vi "Oscilloscope_old.vi"(6 "Slow Control User":string, 9 "notifier in":T4, 10 "queue in":T3) -> ()   [LabVIEW 2012]
uses:
  Oscilloscope/TypeDefs/DataTypes/OscilloscopeState.ctl
  Oscilloscope/TypeDefs/Paths/DataPath.ctl
  <vilib>/Analysis/NI_AALPro.lvlib
  Oscilloscope/TypeDefs/DataTypes/Data.ctl
  TypeDefs/DataTypes/SystemStatus.ctl
  Oscilloscope/TypeDefs/DataTypes/RunInfo.ctl
  Oscilloscope/TypeDefs/DataTypes/UIReferences.ctl
  Oscilloscope/TypeDefs/DataTypes/Measurement.ctl
  Oscilloscope/TypeDefs/DataTypes/Acquisition.ctl
  Oscilloscope/TypeDefs/DataTypes/StopCondition.ctl
  Oscilloscope/TypeDefs/DataTypes/Current.ctl
  Oscilloscope/TypeDefs/DataTypes/DAQConfig.ctl
  <vilib>/Utility/xml.llb/Read From XML File(string).vi
  <vilib>/Analysis/6fits.llb/Remove Outliers (Range).vi
  TypeDefs/QueueNotifier/DataQueue.ctl
  TypeDefs/QueueNotifier/Notifier.ctl
  Oscilloscope/TypeDefs/DataTypes/AcquisitionInfo.ctl
panel:
  in  "SaveToggle":bool caption="Stop Condition"
  in  "Acquisition Info":T1 {"Shaping Amplifier" items=["CR-200-1us", "CR-200-100ns", "", ""]; "Preamplifier" items=["CR-Z-113-1k", "CR-Z-113-5k", "CR-Z-SiPM", ""]}
  out "Acquisition Rate":dbl format="%#.1f"
  in  "Stop":bool
  in  "View TDMS":bool caption="Configure DAQ"
  in  "Trigger Level (V)":dbl=-0.02
  in  "Range (V)":dbl(ring)=2.0 items=["10"=10.0, "5"=5.0, "2"=2.0, "1"=1.0, "0.4"=0.4, "0.2"=0.2, "0.08"=0.08, "0.04"=0.04, "0.02"=0.02, "0.01"=0.01]
  in  "Offset (V)":dbl=-0.5
  out "Acquiring Now?":bool
  out "Active Run?":bool
  out "Time Elapsed (s)":dbl format="%#.1f"
  out "Waveforms Acquired":dbl
  in  "Stop Condition":T2={"Quota"=2000.0, "Duration (S)"=120, "Stop Condition"=FALSE}
  in  "Run Info":bool caption="Configure DAQ"
  out "Signal":waveform(dbl)(graph)
  in  "Measurement (Ch1)":i32(ring)=26 items=["AC RMS"=1, "Amplitude"=2, "Average"=3, "Cycle Average"=4, "Cycle Frequency"=5, "Cycle Period"=6, "Cycle RMS"=7, "DC RMS"=8, "Estimated Number of Bits"=9, "Falling Edges"=10, "Fall Overshoot"=11, "Fall Preshoot"=12, "Frequency"=13, "Fall Crossing Time"=14, "Fall Time"=15, "High"=16, "Low"=17, "Maximum"=18, "Minimum"=19, "Mid"=20, "Negative Duty"=21, "Negative Width"=22, "Positive Duty"=23, "Period"=24, "Phase"=25, "Peak to Peak"=26, "Positive Width"=27, "Rising Edges"=28, "Rise Overshoot"=29, "Rise Preshoot"=30, "Rise Crossing Time"=31, "Rise Time"=32, "Standard Deviation"=33, "Spurious Free Dynamic Range"=34, "Signal to Noise+Distortion"=35, "Signal to Noise"=36, "Total Harmonic Distortion"=37, "Time of Maximum"=38, "Time of Minimum"=39]
  in  "New Run":bool caption="Configure DAQ"
  in  "Export":bool caption="Configure DAQ"
  in  "Exit":bool caption="Configure DAQ"
  in  "Save Run":bool caption="Configure DAQ"
  in  "Settings":bool caption="Configure DAQ"
  in  "Acquire":bool
  out "Preliminary Histogram":cluster{"Y":dbl[], "Y":dbl[]}[](graph)
  # "Shaper Gain"
  # "Self"
  # "Fast"
  # "Solicited"
  # "Standard"
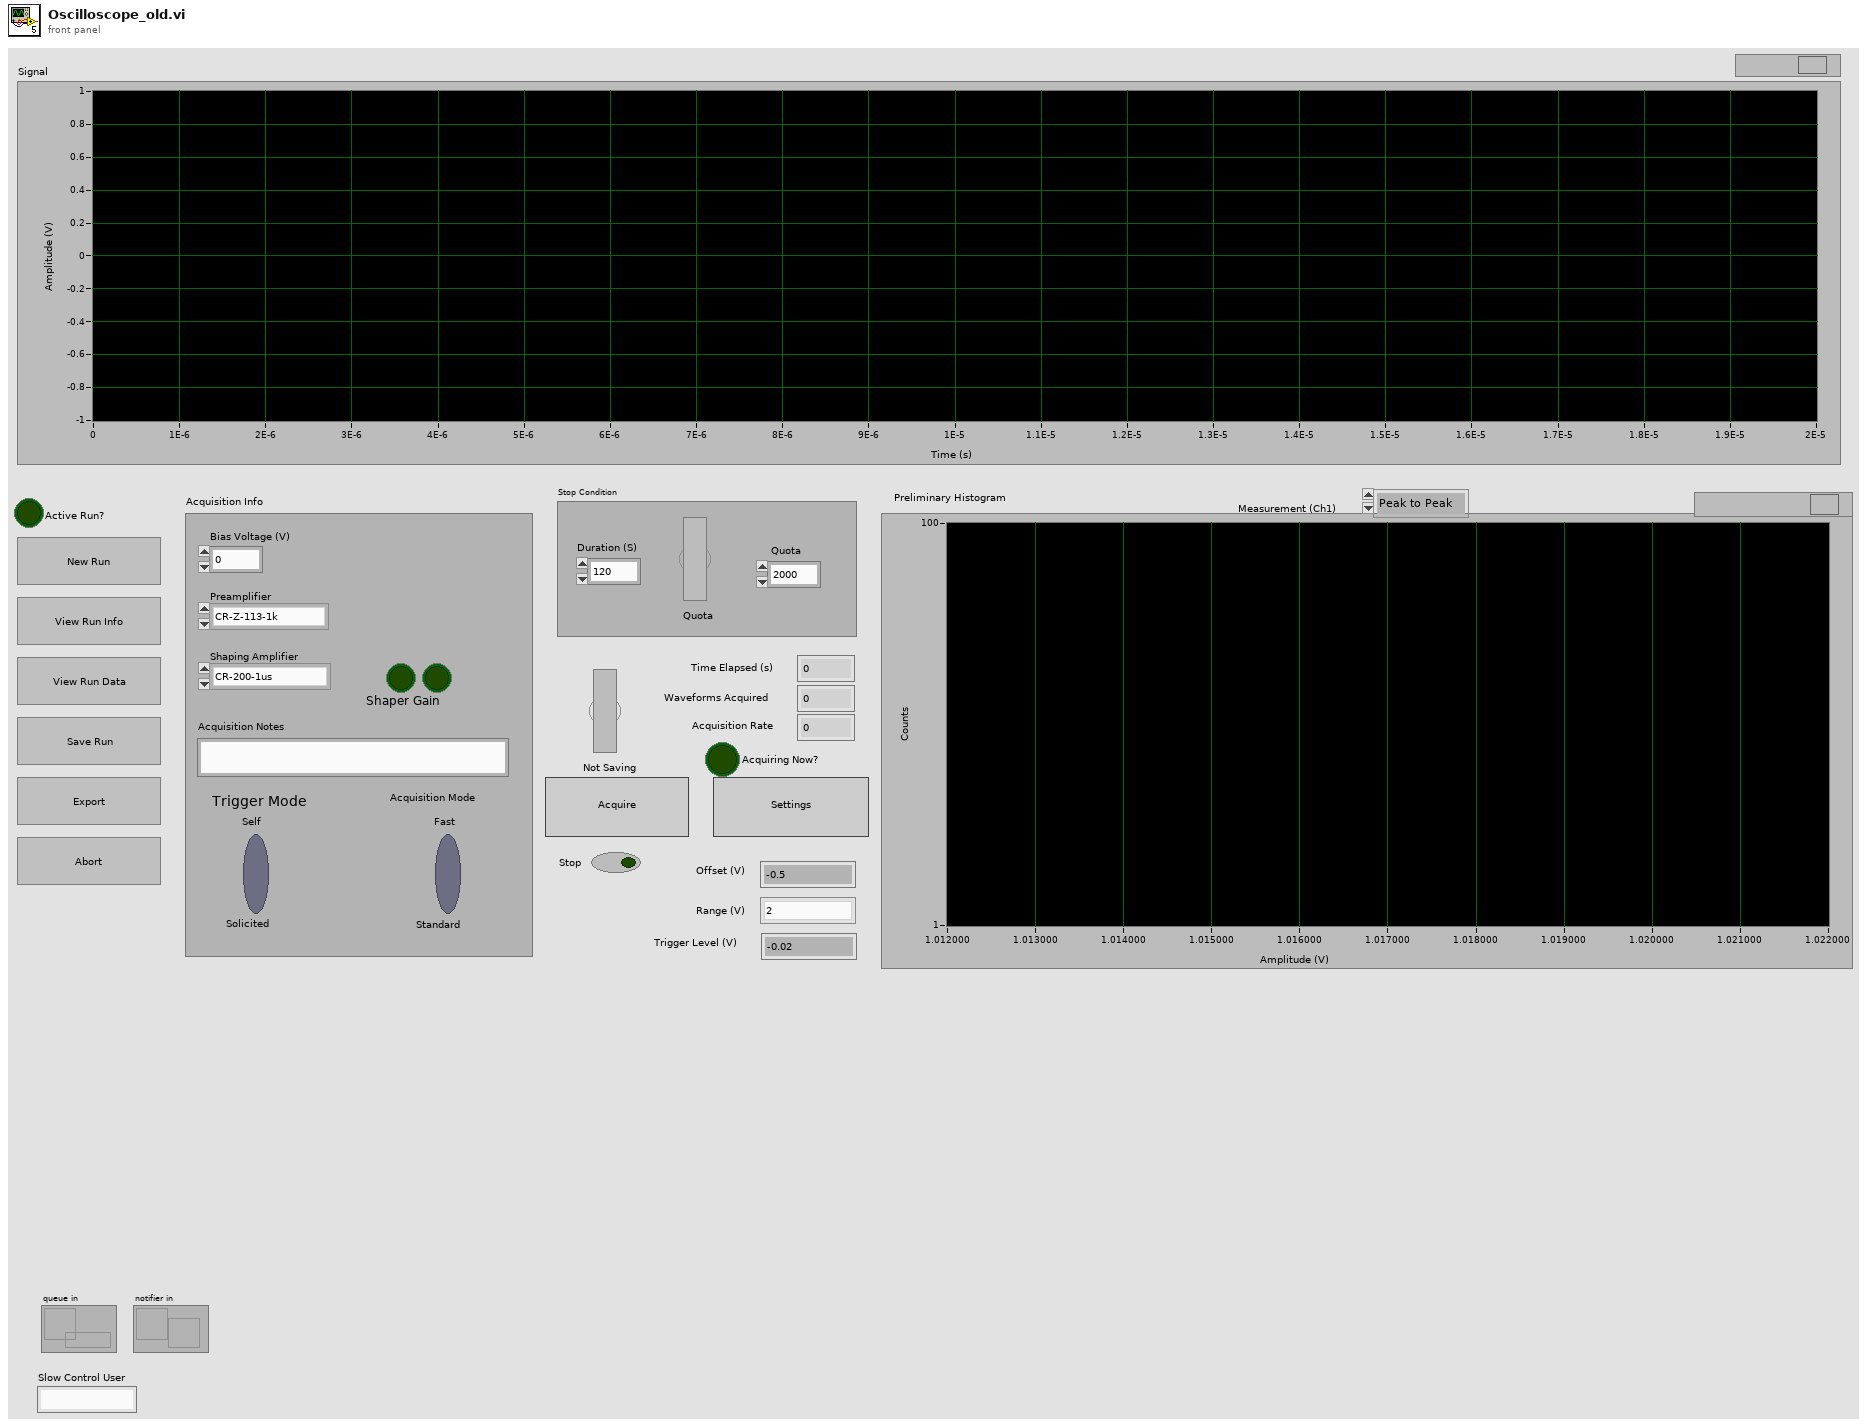
[diagram p1: front panel]
types:
  T1 = typedef "AcquisitionInfo.ctl" = cluster{"Trigger Mode":bool, "Acquisition Mode":bool, "Bias Voltage (V)":dbl, "Preamplifier":u16, "Shaping Amplifier":u16, "Acquisition Notes":string, "1":bool, "2":bool}
  T2 = typedef "StopCondition.ctl" = cluster{"Quota":dbl, "Duration (S)":u16, "Stop Condition":bool}
  T3 = typedef "DataQueue.ctl" = refnum<queue>
  T4 = typedef "Notifier.ctl" = refnum<notifier>
  T5 = typedef "DataPath.ctl" = path
  T6 = typedef "Data.ctl" = cluster{"DAQ Config Data":T7, "Acquisition":T8, "Measurement":T10, "UI References":T11, "Run Info":T12, "System Status":T13, "Acquisition Info":cluster{"Trigger Mode":bool, "Acquisition Mode":bool, "Bias Voltage (V)":dbl, "Preamplifier":u16, "Shaping Amplifier":u16, "Acquisition Notes":string, "1":bool, "2":bool}}
  T7 = typedef "DAQConfig.ctl" = cluster{"Vertical":cluster{"Coupling":i32, "Offset (V)":dbl, "Range (V)":dbl, "Impedance":dbl}, "Horizontal":cluster{"Offset Time":dbl, "Sample Time (S)":dbl, "Sample Points":u32}, "Trigger\n":cluster{"Lower Level (V)":dbl, "Trigger Slope":i32, "Trigger Source":i32}, "Acquisition":cluster{"Trigger Mode":i32, "Initiate Continuously":i32, "Acquire Type":i32, "Acquire Count":i32}, "Channel":i32, "Instrument Handle":i32, "Error":errorcluster, "State":i32}
  T8 = typedef "Acquisition.ctl" = cluster{"Current":T9, "Stop Condition":T2, "Config Needed":bool}
  T9 = typedef "Current.ctl" = cluster{"Acquiring Now?":bool, "Waveforms Acquired":dbl, "Start of Acquisition":timestamp, "Acquisition Name":string}
  T10 = typedef "Measurement.ctl" = cluster{"Waveform":waveform(dbl), "Peak Heights":dbl[], "Acquisition Time":timestamp, "File Path":path, "TDMS File Handle":refnum<k34>}
  T11 = typedef "UIReferences.ctl" = cluster{"Acquire":refnum<vi>, "Configure DAQ":refnum<vi>, "Measurement (Ch1)":refnum<vi>, "Update Needed?":bool, "New Run":refnum<vi>, "Signal":refnum<vi>}
  T12 = typedef "RunInfo.ctl" = cluster{"Active Run?":bool, "Run Notes":string, "User Name":string, "Campaign ID#":string, "Run Name":string, "Start Time":timestamp, "End Time":timestamp}
  T13 = typedef "SystemStatus.ctl" = cluster{"Bias Voltage":dbl, "SiPM Temperature":dbl[], "Slow Control User":string, "LXe":dbl}
  T14 = typedef "OscilloscopeState.ctl" = enum16{"Acquire", "Initialize", "Waiting For Event", "New Run", "Settings", "Update UI", "ViewRunInfo", "Synchronize", "Fast Acquire"}
  T15 = enum8{"Enabled", "Disabled", "Disabled and Grayed Out"}
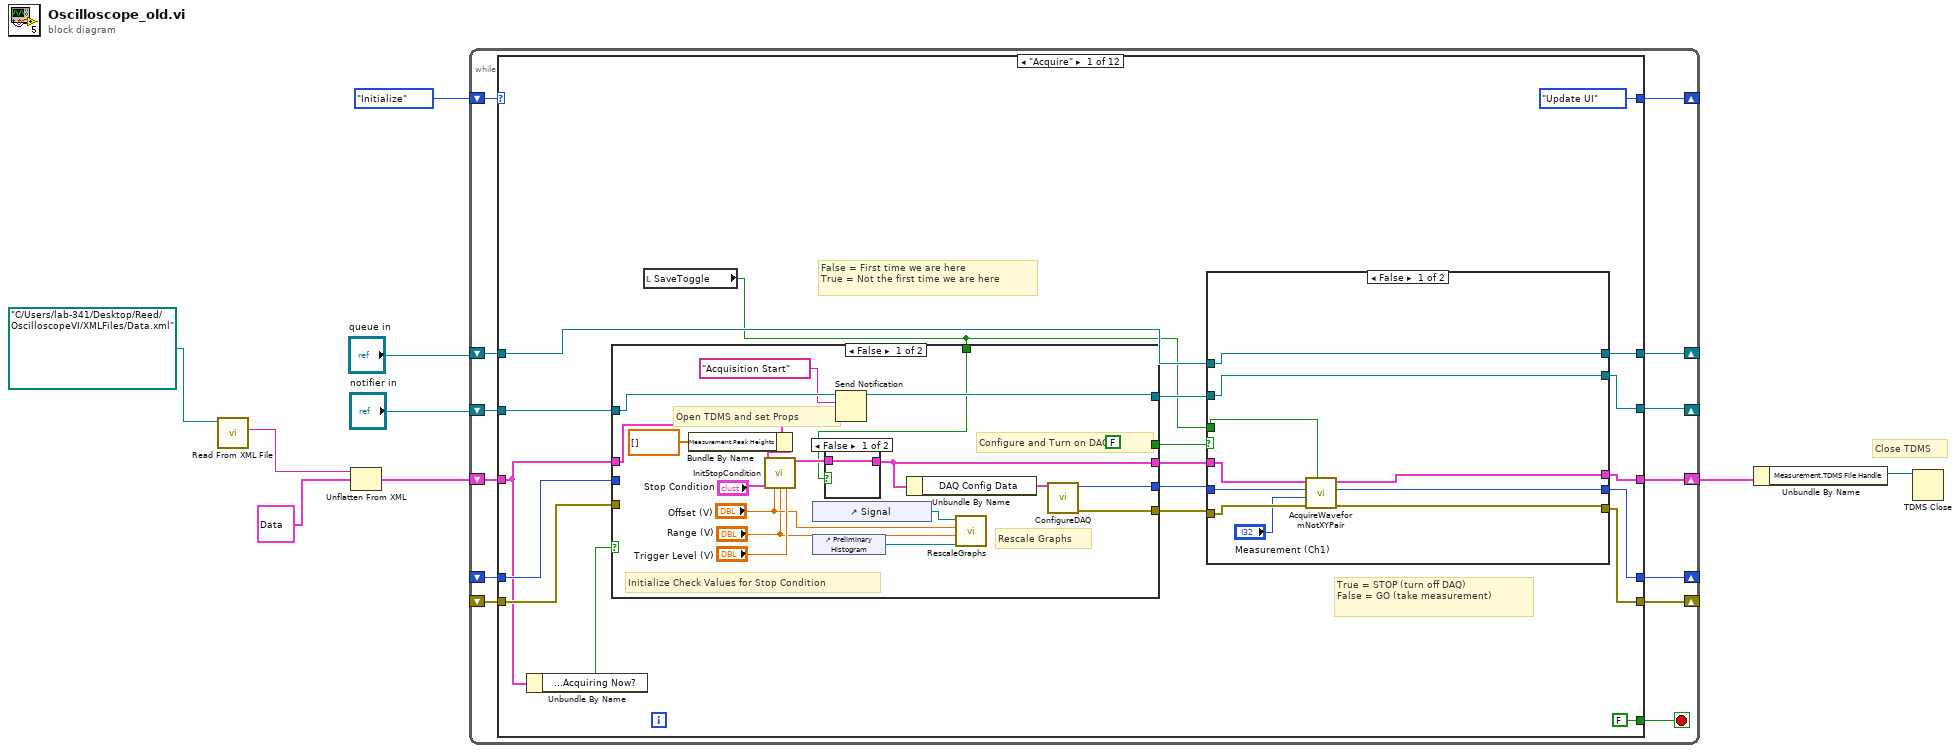
[diagram p0: block diagram]
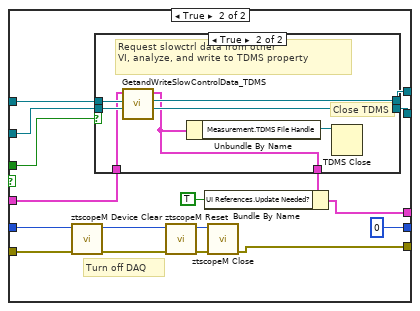
[diagram p2: hidden frame]
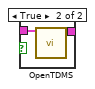
[diagram p4: hidden frame]
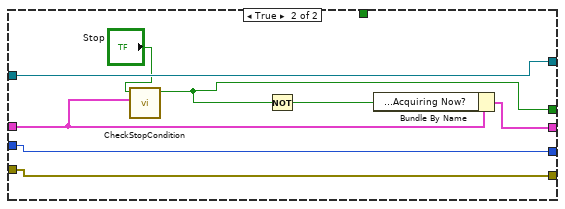
[diagram p5: hidden frame]
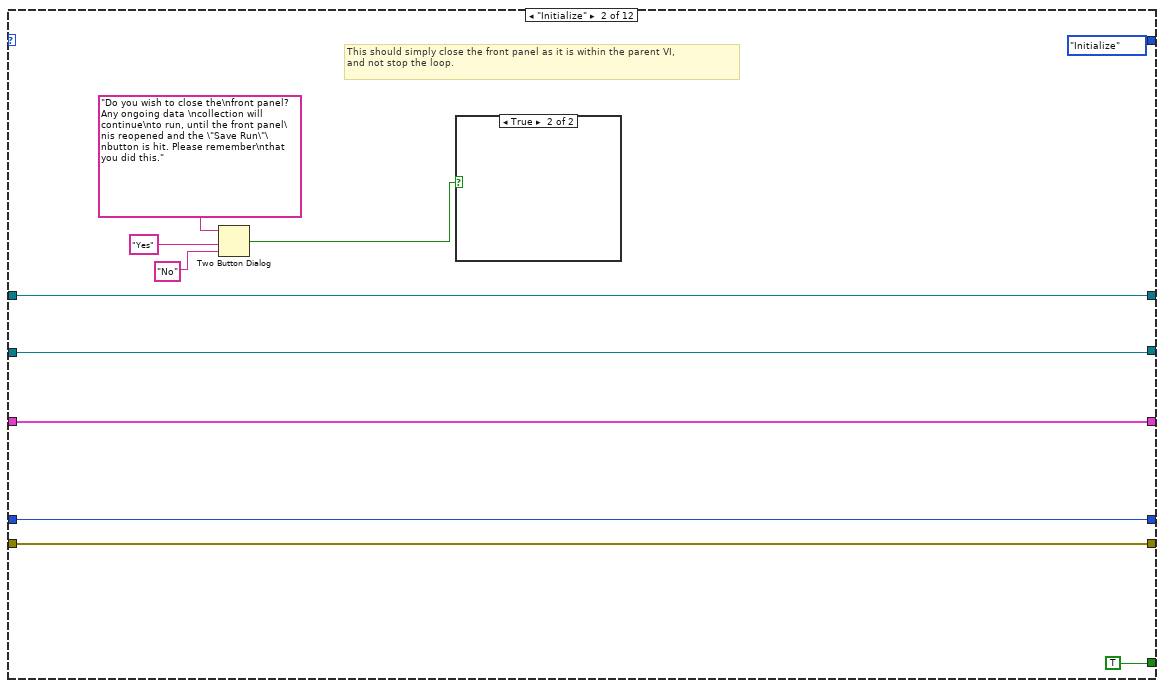
[diagram p6: hidden frame]
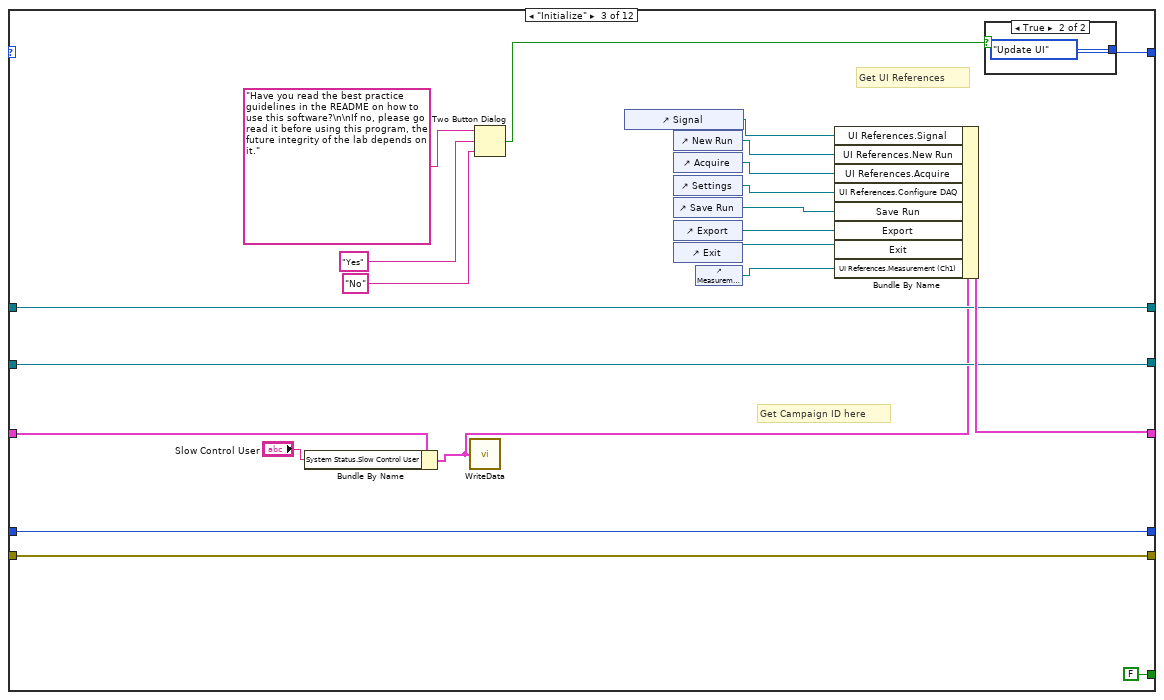
[diagram p8: hidden frame]
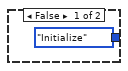
[diagram p9: hidden frame]
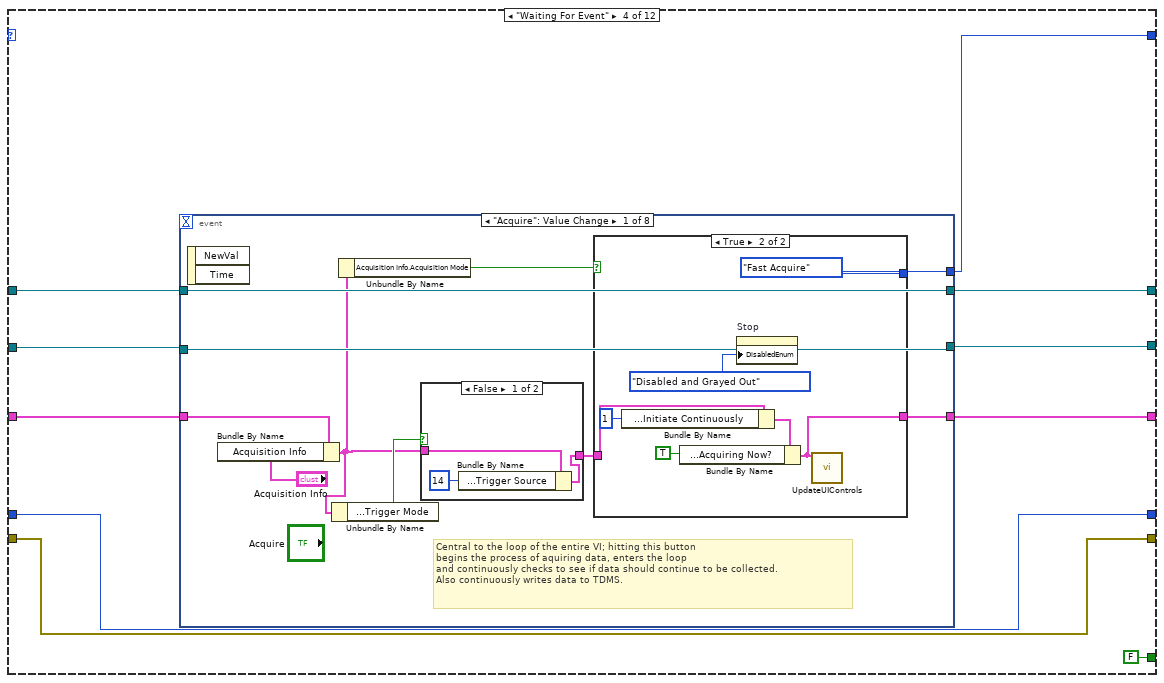
[diagram p10: hidden frame]
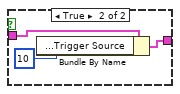
[diagram p11: hidden frame]
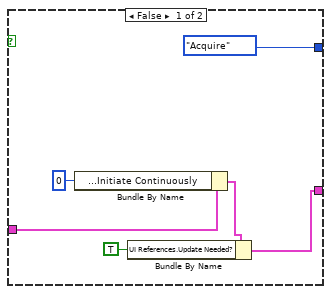
[diagram p12: hidden frame]
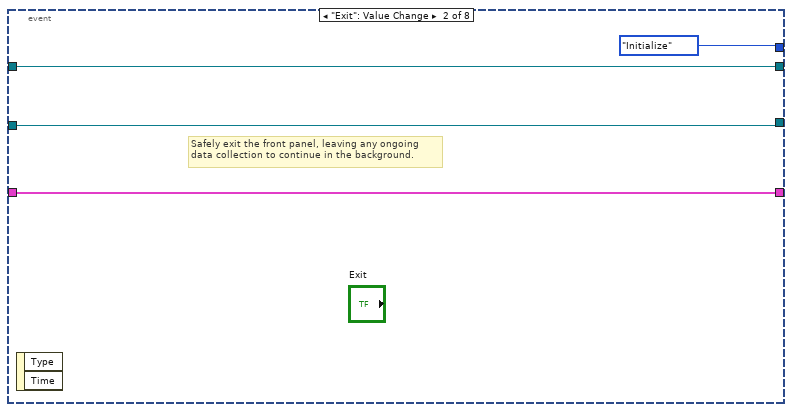
[diagram p13: hidden frame]
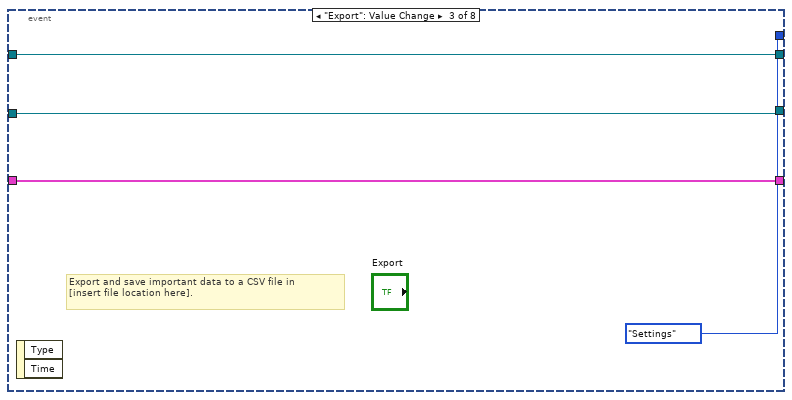
[diagram p14: hidden frame]
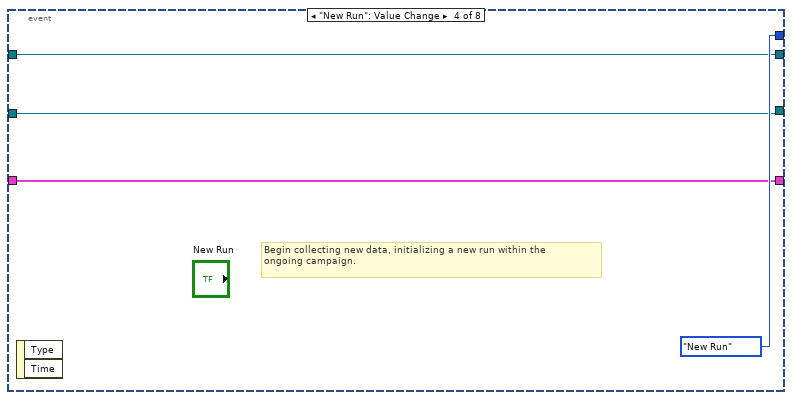
[diagram p15: hidden frame]
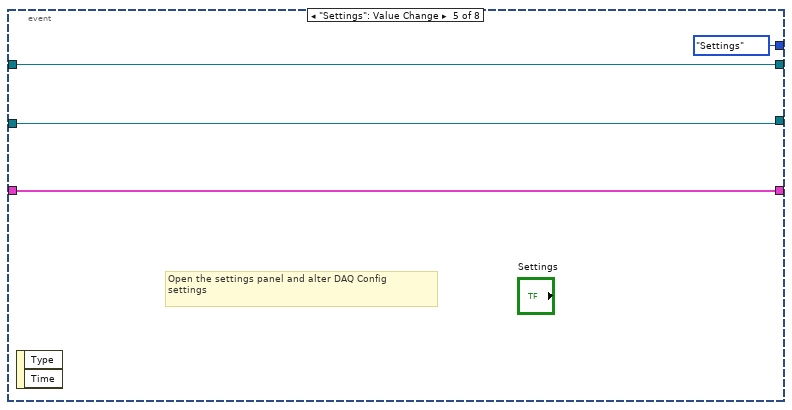
[diagram p16: hidden frame]
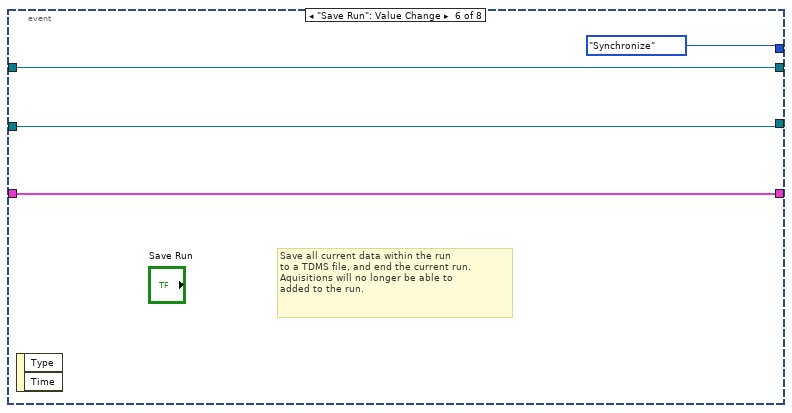
[diagram p17: hidden frame]
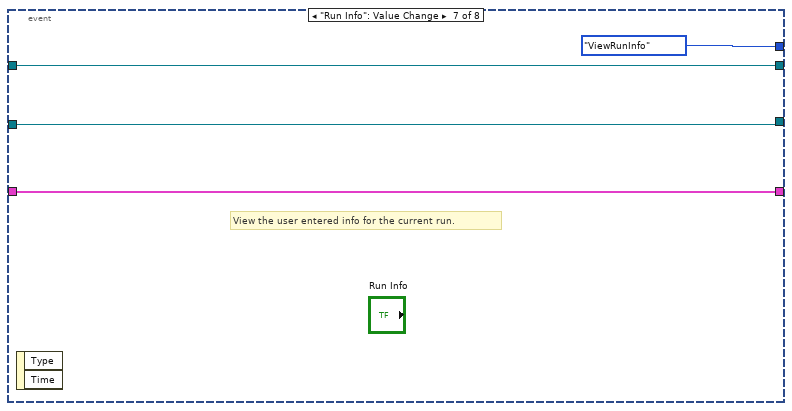
[diagram p18: hidden frame]
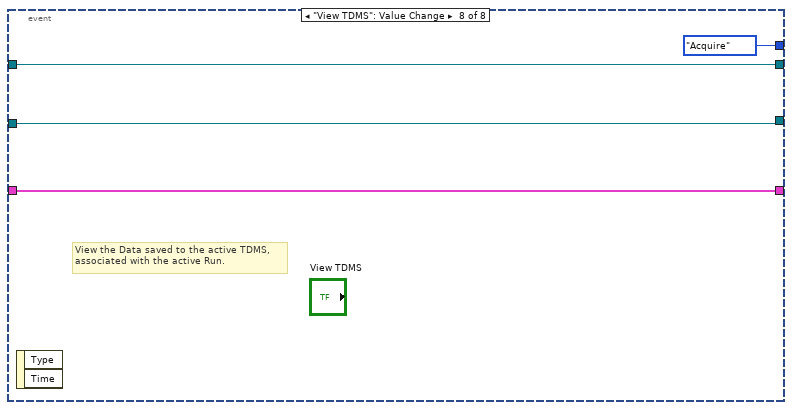
[diagram p19: hidden frame]
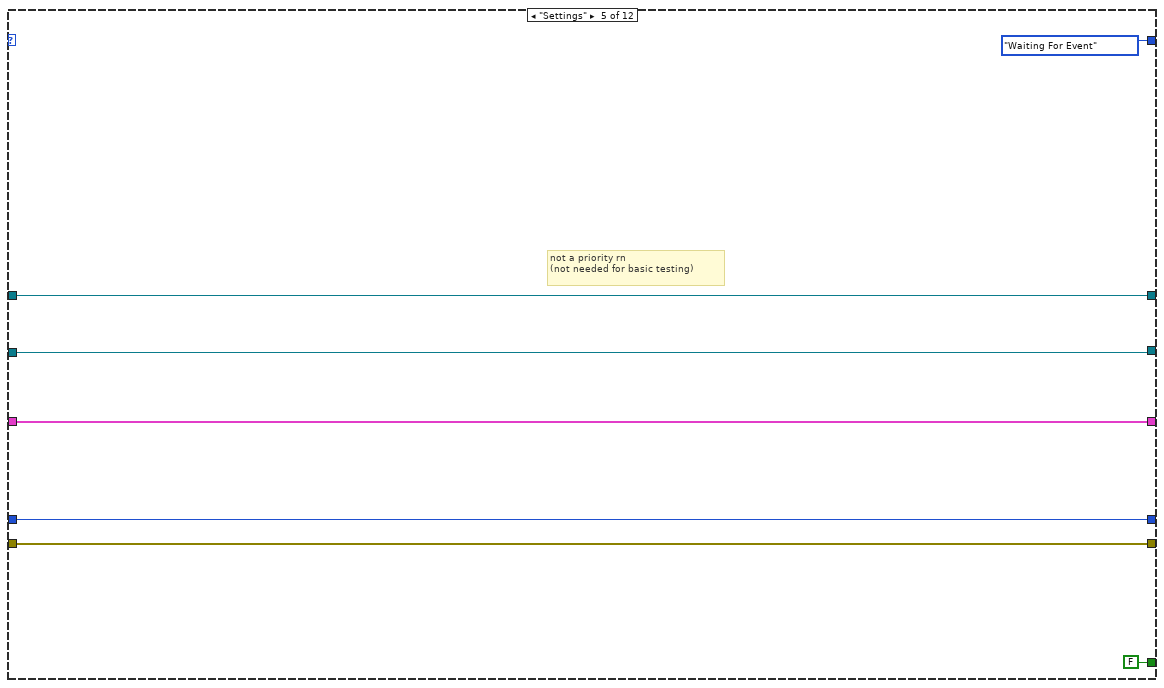
[diagram p20: hidden frame]
diagram:
  # "Close TDMS"
  n1 = call-poly <vilib>:"Read From XML File.vi"("XML File Path"=T5 path "C:/Users/lab-341/Desktop/Reed/OscilloscopeVI/XMLFiles/Data.xml") -> ("XML Elements"=w8:string)  [unwired: 8 in, 2 out]
  n2 = Unflatten From XML(xml string=w8, type=T6 {"DAQ Config Data"={"Vertical"={"Coupling"=1, "Offset (V)"=-0.5, "Range (V)"=2.0, "Impedance"=50.0}, "Horizontal"={"Offset Time"=0.0, "Sample Time (S)"=22.0, "Sample Points"=1000}, "Trigger\n"={"Lower Level (V)"=-0.02, "Trigger Slope"=1, "Trigger Source"=10}, "Acquisition"={"Trigger Mode"=1, "Initiate Continuously"=0, "Acquire Type"=0, "Acquire Count"=0}, "Channel"=0, "Instrument Handle"=0, "Error"={"status"=FALSE, "code"=0, "source"=""}, "State"=1}, "Acquisition"={"Current"={"Acquiring Now?"=FALSE, "Waveforms Acquired"=0.0, "Start of Acquisition"=timestamp(0 s since 1904-01-01), "Acquisition Name"=""}, "Stop Condition"={"Quota"=3000.0, "Duration (S)"=22, "Stop Condition"=FALSE}, "Config Needed"=FALSE}, "Measurement"={"Waveform"={"t0"=timestamp(0 s since 1904-01-01), "dt"=1.0, "Y"=[]}, "Peak Heights"=[], "Acquisition Time"=timestamp(0 s since 1904-01-01), "File Path"=path "", "TDMS File Handle"=refnum}, "UI References"={"Acquire"=refnum, "Configure DAQ"=refnum, "Measurement (Ch1)"=refnum, "Update Needed?"=FALSE, "New Run"=refnum, "Signal"=refnum}, "Run Info"={"Active Run?"=FALSE, "Run Notes"="Enter in notes explaining the purpose of the run and any unusual steps taken in the process. This should make it clear why the data was taken. e.g. \"Measuring LXe scintillation light with Teflon\" or \"Measuring dark pulses to determine SPE gain.\" Concise is good but precise is better.", "User Name"="", "Campaign ID#"="", "Run Name"="", "Start Time"=timestamp(0 s since 1904-01-01), "End Time"=timestamp(0 s since 1904-01-01)}, "System Status"={"Bias Voltage"=0.0, "SiPM Temperature"=[], "Slow Control User"="", "LXe"=0.0}, "Acquisition Info"={"Trigger Mode"=FALSE, "Acquisition Mode"=FALSE, "Bias Voltage (V)"=0.0, "Preamplifier"=0, "Shaping Amplifier"=0, "Acquisition Notes"="", "1"=FALSE, "2"=FALSE}} ("Data")) -> (value=w3:T6)  [unwired: 1 in, 1 out]
  n3 = while {
    shift-right: [w22] -> _
    shift-left: _ -> [w20]
    shift-right: [w19] -> _
    shift-left: _ -> [w21]
    shift-right: [w16] -> w1
    shift-left: w3 -> [w18]
    shift-right: [w14] -> _
    shift-left: OscilloscopeState."Initialize" ("Enum") -> [w17]
    shift-right: [w13] -> _
    shift-left: "notifier in" -> [w10]
    shift-right: [w12] -> _
    shift-left: "queue in" -> [w11]
    stop <- w15 stop-if-true
    n4 = case shown="\"Acquire\"" w17 {
      tunnel: [w38 w119 w139 w152 w216 w227 w261 w277 w315 w333 w343 w371] -> w19
      tunnel: [w37 w118 w138 w151 w215 w226 w260 w276 w314 w332 w342 w370] -> w22
      tunnel: w21 -> [w32 w119 w139 w152 w216 w227 w261 w277 w315 w333 w343 w371]
      tunnel: w20 -> [w31 w118 w138 w151 w215 w226 w260 w276 w314 w332 w342 w370]
      tunnel: w18 -> [w24 w113 w122 w144 w217 w223 w251 w266 w307 w329 w339 w359]
      tunnel: [OscilloscopeState."Update UI" ("Enum") OscilloscopeState."Initialize" ("Enum") w141 w145 OscilloscopeState."Waiting For Event" ("Enum") OscilloscopeState."Update UI" ("Enum") OscilloscopeState."Waiting For Event" ("Enum") OscilloscopeState."Update UI" ("Enum") w319 OscilloscopeState."Waiting For Event" ("Enum") OscilloscopeState."Waiting For Event" ("Enum") OscilloscopeState."Update UI" ("Enum")] -> w14
      tunnel: [w36 w113 w140 w153 w217 w221 w262 w270 w316 w329 w339 w348] -> w16
      tunnel: [FALSE TRUE FALSE FALSE FALSE FALSE FALSE FALSE FALSE FALSE FALSE FALSE] -> w15
      tunnel: [w27 w114 w124 w149 w211 w218 w256 w267 w310 w334 w344 w349] -> w13
      tunnel: w11 -> [w25 w115 w125 w148 w212 w219 w257 w268 w311 w335 w345 w352]
      tunnel: [w29 w115 w125 w147 w212 w219 w257 w268 w311 w335 w345 w351] -> w12
      tunnel: w10 -> [w26 w114 w124 w146 w211 w218 w256 w267 w310 w334 w344 w354]
      frame "Acquire" {
        # "False = First time we are here\nTrue = Not the first time we are here"
        # "True = STOP (turn off DAQ)\nFalse = GO (take measurement)"
        n5 = Unbundle By Name(w24) -> ("Acquisition.Current.Acquiring Now?"=w41:bool)
        n6 = local read "SaveToggle"() -> (w23:bool)
        n7 = case shown="False" w41 {
          tunnel: w24 -> [w80 w108]
          tunnel: [w89 w107] -> w35
          tunnel: [FALSE w102] -> w39
          tunnel: [w96 w105] -> w34
          tunnel: [w95 w104] -> w33
          tunnel: w32 -> [_ w105]
          tunnel: w31 -> [_ w104]
          tunnel: w26 -> [w94 w103]
          tunnel: [w93 w103] -> w28
          tunnel: w23 -> [w79 _]
          frame False {
            # "Rescale Graphs"
            # "Open TDMS and set Props"
            # "Configure and Turn on DAQ"
            # "Initialize Check Values for Stop Condition"
            n8 = Bundle By Name(cluster=w80, "Measurement.Peak Heights"=dbl[] []) -> (w81:T6)
            n9 = call "InitStopCondition.vi"("Data"=w81, "Stop Condition"="Stop Condition", "Offset (V)"="Offset (V)", "Range (V)"="Range (V)", "Trigger Level (V)"="Trigger Level (V)") -> ("Data Out"=w88:T6)  [unwired: 10 in]
            n10 = control-ref of="Signal"() -> (w84:refnum<vi>)
            n11 = control-ref of="Preliminary Histogram"() -> (w83:refnum<vi>)
            n12 = case shown="False" w79 {
              tunnel: [w98 w100] -> w89
              tunnel: w88 -> [w98 w99]
              frame False {
              }
              frame True {
                n13 = call "OpenTDMS.vi"("Data In"=w99) -> ("Data Out"=w100:T6)  [unwired: 9 in]
              }
            }
            n14 = Send Notification(notification="Acquisition Start", notifier=w94) -> (notifier out=w93:T4)  [unwired: 1 in, 1 out]
            n15 = Unbundle By Name(w89) -> ("DAQ Config Data"=w90:T7)
            n16 = call "RescaleGraphs.vi"("WaveformGraph in"=w84, "Offset (V) 3"="Offset (V)", "Range (V) 3"="Range (V)", "Preliminary Histogram"=w83) -> ()  [unwired: 6 in]
            n17 = call "ConfigureDAQ.vi"("DAQ Config Data"=w90) -> ("error out"=w95:errorcluster, "Instrument Handle Out"=w96:i32)  [unwired: 9 in]
          }
          frame True {
            n18 = call "CheckStopCondition.vi"("Data"=w108, "Stop"="Stop") -> ("f"=w102:bool)  [unwired: 9 in]
            n19 = Not(x=w102) -> (.not. x?=w106:bool)
            n20 = Bundle By Name(cluster=w108, "Acquisition.Current.Acquiring Now?"=w106) -> (w107:T6)
          }
        }
        n21 = case shown="False" w39 {
          tunnel: w34 -> [w51 w65]
          tunnel: w33 -> [w50 w64]
          tunnel: [w48 0 ("Instrument Handle Out out")] -> w38
          tunnel: [w49 w63] -> w37
          tunnel: w35 -> [w46 w58]
          tunnel: [w45 w54] -> w36
          tunnel: [w44 w57] -> w29
          tunnel: w25 -> [w44 w60]
          tunnel: w28 -> [w43 w59]
          tunnel: [w43 w56] -> w27
          tunnel: w23 -> [w42 w52]
          frame False {
            n22 = call "AcquireWaveformNotXYPair.vi"(7:w42, "error in (no error)"=w50, "Measurement (Ch1)"="Measurement (Ch1)", "Instrument Handle In"=w51, "Data in"=w46) -> ("error out"=w49:errorcluster, "Instrument Handle Out"=w48:i32, "Data out"=w45:T6)  [unwired: 4 in]
          }
          frame True {
            # "Turn off DAQ"
            n23 = call <instrlib>:"ztscopeM Device Clear.vi"("error in"=w64, "Instrument Handle In"=w65) -> ("error out"=w66:errorcluster, "Instrument Handle Out"=w68:i32)  [unwired: 8 in]
            n24 = case shown="True" w52 {
              tunnel: w60 -> [w71 w78]
              tunnel: w59 -> [w70 w77]
              tunnel: w58 -> [w69 w76]
              tunnel: [w71 w75] -> w57
              tunnel: [w70 w74] -> w56
              tunnel: [w69 w72] -> w55
              frame False {
              }
              frame True {
                # "Request slowctrl data from other\nVI, analyze, and write to TDMS property"
                # "Close TDMS"
                n25 = call "GetandWriteSlowControlData_TDMS.vi"("notifier in"=w77, "queue in"=w78, "Data In"=w76) -> ("notifier out"=w74:T4, "queue out"=w75:T3, "Data Out"=w72:T6)  [unwired: 6 in]
                n26 = Unbundle By Name(w72) -> ("Measurement.TDMS File Handle"=w73:refnum<k34>)
                n27 = TDMS Close(11:w73) -> ()  [unwired: 1 in, 2 out]
              }
            }
            n28 = call <instrlib>:"ztscopeM Reset.vi"("error in"=w66, "Instrument Handle In"=w68) -> ("error out"=w67:errorcluster, "Instrument Handle Out"=w62:i32)  [unwired: 8 in]
            n29 = Bundle By Name(cluster=w55, "UI References.Update Needed?"=TRUE) -> (w54:T6)
            n30 = call <instrlib>:"ztscopeM Close.vi"("error in"=w67, "Instrument Handle In"=w62) -> ("error out"=w63:errorcluster)  [unwired: 9 in]
          }
        }
      }
      frame "Initialize" {
        # "This should simply close the front panel as it is within the parent VI,\nand not stop the loop."
        n31 = Two Button Dialog(message="Do you wish to close the\nfront panel? Any ongoing data \ncollection will continue\nto run, until the front panel\nis reopened and the \"Save Run\"\nbutton is hit. Please remember\nthat you did this.", 1:"No" ("F button name (\"Cancel\")"), 2:"Yes" ("T button name (\"OK\")")) -> (T button?=w109:bool)
        n32 = case shown="True" w109 {
          frame False {
          }
          frame True {
          }
        }
      }
      frame "Initialize" {
        # "Get Campaign ID here"
        # "Get UI References"
        n33 = Bundle By Name(cluster=w122, "System Status.Slow Control User"="Slow Control User") -> (w120:T6)
        n34 = call "WriteData.vi"("Data"=w120) -> ()  [unwired: 6 in]
        n35 = Two Button Dialog(message="Have you read the best practice guidelines in the README on how to use this software?\n\nIf no, please go read it before using this program, the future integrity of the lab depends on it.", 1:"No" ("F button name (\"Cancel\")"), 2:"Yes" ("T button name (\"OK\")")) -> (T button?=w132:bool)
        n36 = control-ref of="Signal"() -> (w123:refnum<vi>)
        n37 = control-ref of="New Run"() -> (w131:refnum<vi>)
        n38 = control-ref of="Acquire"() -> (w130:refnum<vi>)
        n39 = control-ref of="Settings"() -> (w129:refnum<vi>)
        n40 = control-ref of="Save Run"() -> (w128:refnum<vi>)
        n41 = control-ref of="Export"() -> (w127:refnum<vi>)
        n42 = control-ref of="Exit"() -> (w126:refnum<vi>)
        n43 = control-ref of="Measurement (Ch1)"() -> (w137:refnum<vi>)
        n44 = Bundle By Name(cluster=w120, "UI References.Signal"=w123, "UI References.New Run"=w131, "UI References.Acquire"=w130, "UI References.Configure DAQ"=w129, "Save Run"=w128, "Export"=w127, "Exit"=w126, "UI References.Measurement (Ch1)"=w137) -> (w140:T6)
        n45 = case shown="True" w132 {
          tunnel: [OscilloscopeState."Initialize" ("Enum") OscilloscopeState."Update UI" ("Enum")] -> w141
          frame False {
          }
          frame True {
          }
        }
      }
      frame "Waiting For Event" {
        n46 = event shown="[0] \"Acquire\": Value Change" {
          selector: _ -> [_ _ _ _ _ _ _ _]
          dyn-events: _ -> [_ _ _ _ _ _ _ _]
          timeout: _ -> [_ _ _ _ _ _ _ _]
          tunnel: [w159 OscilloscopeState."Initialize" ("Enum") OscilloscopeState."Settings" ("Enum") OscilloscopeState."New Run" ("Enum") OscilloscopeState."Settings" ("Enum") OscilloscopeState."Synchronize" ("Enum") OscilloscopeState."ViewRunInfo" ("Enum") OscilloscopeState."Acquire" ("Enum")] -> w145
          tunnel: w144 -> [w160 w183 w187 w191 w195 w199 w203 w207]
          tunnel: [w158 w183 w187 w191 w195 w199 w203 w207] -> w153
          tunnel: w146 -> [w162 w184 w188 w192 w196 w200 w204 w210]
          tunnel: [w162 w184 w188 w192 w196 w200 w204 w210] -> w149
          tunnel: [w163 w185 w189 w193 w197 w201 w205 w209] -> w147
          tunnel: w148 -> [w163 w185 w189 w193 w197 w201 w205 w209]
          event "Acquire": Value Change {
            # "Central to the loop of the entire VI; hitting this button\nbegins the process of aquiring data, enters the loop \nand continuously checks to see if data should continue to be collected. \nAlso continuously writes data to TDMS."
            n47 = event-data() -> ()  [unwired: 1 in, 2 out]
            n48 = Bundle By Name(cluster=w160, "Acquisition Info"="Acquisition Info") -> (w155:T6)
            n49 = Unbundle By Name(w155) -> ("Acquisition Info.Trigger Mode"=w156:bool)
            n50 = Unbundle By Name(w155) -> ("Acquisition Info.Acquisition Mode"=w157:bool)
            n51 = case shown="False" w156 {
              tunnel: w155 -> [w165 w168]
              tunnel: [w164 w167] -> w154
              frame False {
                n52 = Bundle By Name(cluster=w165, "DAQ Config Data.Trigger.Trigger Source"=14 ("DAQ Config Data.Trigger\n.Trigger Source")) -> (w164:T6)
              }
              frame True {
                n53 = Bundle By Name(cluster=w168, "DAQ Config Data.Trigger.Trigger Source"=10 ("DAQ Config Data.Trigger\n.Trigger Source")) -> (w167:T6)
              }
            }
            n54 = case shown="True" w157 {
              tunnel: [OscilloscopeState."Acquire" ("t") OscilloscopeState."Fast Acquire" ("t")] -> w159
              tunnel: w154 -> [w172 w179]
              tunnel: [w173 w180] -> w158
              frame False {
                n55 = Bundle By Name(cluster=w172, "DAQ Config Data.Acquisition.Initiate Continuously"=0) -> (w171:T6)
                n56 = Bundle By Name(cluster=w171, "UI References.Update Needed?"=TRUE) -> (w173:T6)
              }
              frame True {
                n57 = Bundle By Name(cluster=w179, "DAQ Config Data.Acquisition.Initiate Continuously"=1) -> (w178:T6)
                n58 = Bundle By Name(cluster=w178, "Acquisition.Current.Acquiring Now?"=TRUE) -> (w180:T6)
                n59 = property on="Stop" class="Bool"("DisabledEnum"=T15."Disabled and Grayed Out" ("Disabled")) -> ()  [unwired: 2 in, 2 out]
                n60 = call "UpdateUIControls.vi"("Data"=w180) -> ()  [unwired: 11 in]
              }
            }
          }
          event "Exit": Value Change {
            # "Safely exit the front panel, leaving any ongoing \ndata collection to continue in the background."
            n61 = event-data() -> ()  [unwired: 1 in, 2 out]
          }
          event "Export": Value Change {
            # "Export and save important data to a CSV file in\n[insert file location here]."
            n62 = event-data() -> ()  [unwired: 1 in, 2 out]
          }
          event "New Run": Value Change {
            # "Begin collecting new data, initializing a new run within the \nongoing campaign."
            n63 = event-data() -> ()  [unwired: 1 in, 2 out]
          }
          event "Settings": Value Change {
            # "Open the settings panel and alter DAQ Config\nsettings"
            n64 = event-data() -> ()  [unwired: 1 in, 2 out]
          }
          event "Save Run": Value Change {
            # "Save all current data within the run\nto a TDMS file, and end the current run.\nAquisitions will no longer be able to \nadded to the run."
            n65 = event-data() -> ()  [unwired: 1 in, 2 out]
          }
          event "Run Info": Value Change {
            # "View the user entered info for the current run."
            n66 = event-data() -> ()  [unwired: 1 in, 2 out]
          }
          event "View TDMS": Value Change {
            # "View the Data saved to the active TDMS,\nassociated with the active Run."
            n67 = event-data() -> ()  [unwired: 1 in, 2 out]
          }
        }
      }
      frame "Settings" {
        # "not a priority rn \n(not needed for basic testing)"
      }
      frame "New Run" {
        # "This VI still needs to fix Config New Run subVI. Need to get Campaign ID# from other\nLabVIEW VI and figure something out for  generating a Run ID#. Also need to make\nsure that TDMS file definitely gets flushed."
        n68 = flat-sequence {
          tunnel: [w229] -> w224
          tunnel: w223 -> [w228]
          tunnel: [w228] -> w222
          tunnel: w224 -> [w238]
          tunnel: w222 -> [w237]
          tunnel: [w236] -> w221
          frame #0 {
            n69 = Unbundle By Name(w228) -> ("Run Info.Active Run?"=w230:bool)
            n70 = case shown="True" w230 {
              tunnel: [TRUE ("T button?") w234] -> w229
              frame False {
              }
              frame True {
                n71 = Two Button Dialog(message="There is currently an active run in the local\nfiles. If you create a new run now, it will\noverwrite the existing data. Cancel and press\nSave Run to finish the current Run and\ncompile the measurement files to permanent\nstorage in HDF5 files.", 1:"Cancel" ("F button name (\"Cancel\")"), 2:"Continue" ("T button name (\"OK\")")) -> (T button?=w234:bool)
              }
            }
          }
          frame #1 {
            n72 = case shown="True" w238 {
              tunnel: w237 -> [w239 w243]
              tunnel: [w239 w240] -> w236
              frame False {
              }
              frame True {
                # "Config New Run"
                n73 = call "NewRunDialog.vi"() -> ("Run Info Out"=w242:T12)  [unwired: 10 in]
                n74 = Bundle By Name(cluster=w243, "Run Info"=w242, "UI References.Update Needed?"=TRUE) -> (w241:T6)
                n75 = call "ReadData.vi"() -> ("Data"=w246:T6)  [unwired: 8 in]
                n76 = Bundle By Name(cluster=w246, "Run Info"=w242) -> (w245:T6)
                n77 = call "WriteData.vi"("Data"=w245) -> ()  [unwired: 6 in]
                n78 = call "NewTDMSFile.vi"("Data In"=w241) -> ("Data Out"=w240:T6)  [unwired: 10 in]
              }
            }
          }
        }
      }
      frame "Settings" {
        n79 = local read "Trigger Level (V)"() -> (w247:dbl)
        n80 = local read "Offset (V)"() -> (w249:dbl)
        n81 = local read "Range (V)"() -> (w248:dbl)
        n82 = Bundle By Name(cluster=w251, "DAQ Config Data.Vertical.Offset (V)"=w249, "DAQ Config Data.Vertical.Range (V)"=w248, "DAQ Config Data.Trigger.Lower Level (V)"=w247) -> (w250:T6)
        n83 = Unbundle By Name(w250) -> ("DAQ Config Data"=w263:T7)
        n84 = call "SettingsDialog.vi"("DAQ Config In"=w263) -> ("DAQ Config Out"=w255:T7)  [unwired: 8 in]
        n85 = Unbundle By Name(w255) -> ("Vertical.Offset (V)"=w254:dbl, "Vertical.Range (V)"=w253:dbl, "Trigger.Lower Level (V)"=w252:dbl)
        n86 = local write "Offset (V)"(w254) -> ()
        n87 = local write "Range (V)"(w253) -> ()
        n88 = local write "Trigger Level (V)"(w252) -> ()
        n89 = call "ReadData.vi"() -> ("Data"=w265:T6)  [unwired: 8 in]
        n90 = Bundle By Name(cluster=w265, "DAQ Config Data"=w255) -> (w264:T6)
        n91 = Bundle By Name(cluster=w250, "DAQ Config Data"=w255) -> (w262:T6)
        n92 = call "WriteData.vi"("Data"=w264) -> ()  [unwired: 6 in]
      }
      frame "Synchronize" {
        n93 = Two Button Dialog(message="Pressing continue will compile all waveforms in the current run from TDMS to HDF5 and flush the TDMS files. This will end the current run, so you will no longer be able to append measurements to it. The purpose of the run system is to group data that should be analyzed, plotted, and fit together. To avoid over-fragmenting of data that would have to be re-collected later, please follow the guidelines in the README for when to start a New Run and avoid using two or more Runs where one would suffice.", 1:"Cancel" ("F button name (\"Cancel\")"), 2:"Continue" ("T button name (\"OK\")")) -> (T button?=w272:bool)
        n94 = case shown="True" w272 {
          tunnel: w266 -> [_ w284]
          tunnel: w266 -> [w278 w281]
          tunnel: [w278 w280] -> w270
          frame False {
          }
          frame True {
            n95 = Bundle By Name(cluster=w281, "Run Info.Active Run?"=FALSE, "UI References.Update Needed?"=TRUE) -> (w280:T6)
            n96 = flat-sequence {
              tunnel: w284 -> [w285]
              tunnel: [w285] -> w279
              tunnel: w279 -> [w286]
              frame #0 {
                n97 = call "SaveRunUpdateXML.vi"("Data"=w285) -> ()  [unwired: 11 in]
              }
              frame #1 {
                n98 = Unbundle By Name(w286) -> ("Measurement.File Path"=w287:path)
                n99 = TDMS Defragment(7:w287) -> ()  [unwired: 1 in, 1 out]
              }
              frame #2 {
                n100 = call <vilib>:"System Exec.vi"("run minimized? (F)"=FALSE, "command line"="python C:\\Users\\lab-341\\Desktop\\Reed\\OscilloscopeVI\\PythonScripts\\TDMStoHDF5.txt") -> ()  [unwired: 6 in, 4 out]
              }
            }
          }
        }
      }
      frame "Update UI" {
        # "Reset Indicator"
        n101 = Unbundle By Name(w307) -> ("DAQ Config Data.Horizontal.Offset Time"=w303:dbl, "Measurement.Waveform"=→"Signal":waveform(dbl), "Measurement.Peak Heights"=w291:dbl[], "DAQ Config Data.Vertical.Range (V)"=w294:dbl, "DAQ Config Data.Vertical.Offset (V)"=w295:dbl, "Acquisition.Current.Waveforms Acquired"=w299:dbl, "Acquisition.Current.Start of Acquisition"=w301:timestamp)
        "Waveforms Acquired" <- w299
        n102 = Unbundle By Name(w307) -> ("Run Info.Active Run?"=→"Active Run?":bool)
        n103 = Get Date/Time In Seconds() -> (seconds since 1Jan1904=w300:timestamp)
        n104 = Negate(x=w303) -> (-x=w302:dbl)
        n105 = Subtract(x=w300, y=w301) -> (x-y=w306:dbl)
        "Time Elapsed (s)" <- w306
        n106 = Subtract(x=w295, y=w294) -> (x-y=w293:dbl)
        n107 = property on="Signal" class="WFGraph (strict)"("XScale.Offset"=w302) -> ()  [unwired: 2 in, 2 out]
        n108 = Add(x=w294, y=w295) -> (x+y=w296:dbl)
        n109 = Unbundle By Name(w307) -> ("UI References.Update Needed?"=w317:bool)
        n110 = Build Array(w296, w293) -> (w292:dbl[])
        n111 = call-poly <vilib>:"Remove Outliers.vi"("Y"=w291, "X"=w291, "Range"=w292) -> ("Y Out"=w297:dbl[])  [unwired: 8 in, 4 out]
        n112 = Divide(x=w299, y=w306) -> (x/y=→"Acquisition Rate":dbl)
        n113 = call <vilib>:"General Histogram.vi"("X"=w297, "# bins"=1000) -> ("Histogram"=w298:i32[], "Axis"=w322:dbl[])  [unwired: 9 in, 3 out]
        n114 = case shown="True" w317 {
          tunnel: w307 -> [w326 w327]
          tunnel: [w326 w327] -> w309
          frame False {
            # "Reduce \nOverhead"
          }
          frame True {
            # "Enable/Disable\nControls"
            n115 = call "UpdateUIControls.vi"("Data"=w327) -> ()  [unwired: 11 in]
          }
        }
        n116 = call "Convert to Dynamic Data4"("Array"=w298) -> ("Dynamic Data Type"=w320:dynamicdata)  [unwired: 3 in]
        n117 = call "Convert to Dynamic Data3"("Array"=w322) -> ("Dynamic Data Type"=w321:dynamicdata)  [unwired: 3 in]
        n118 = call "Temporary Histogram Graph"("Y Input"=w320, "X Input"=w321) -> ("XY Graph"=→"Preliminary Histogram":cluster{"Y":dbl[], "Y":dbl[]}[])  [unwired: 3 in, 6 out]
        n119 = Unbundle By Name(w309) -> ("Acquisition.Current.Acquiring Now?"=w312:bool)
        "Acquiring Now?" <- w312
        n120 = case shown="False" w312 {
          tunnel: [OscilloscopeState."Waiting For Event" ("Enum") OscilloscopeState."Acquire" ("Enum")] -> w319
          frame False {
          }
          frame True {
          }
        }
        n121 = Bundle By Name(cluster=w309, "UI References.Update Needed?"=FALSE) -> (w316:T6)
      }
      frame "ViewRunInfo" {
        n122 = Unbundle By Name(w329) -> ("Acquisition.Current.Acquiring Now?"=w328:bool)
        n123 = case shown="False" w328 {
          tunnel: w329 -> [w336 _]
          frame False {
            n124 = Unbundle By Name(w336) -> ("Run Info"=w337:T12)
            n125 = call "ViewRunInfo.vi"("Run Info In"=w337) -> ()  [unwired: 11 in]
          }
          frame True {
          }
        }
      }
      frame "Acquire" {
        n126 = Unbundle By Name(w339) -> ("Acquisition.Current.Acquiring Now?"=w338:bool)
        n127 = case shown="False" w338 {
          frame False {
            n128 = call <vilib>:"TDMS - File Viewer.vi"("file path"=path "C:/Users/lab-341/Desktop/Reed/OscilloscopeVI/pulses.tdms") -> ()  [unwired: 5 in, 2 out]
          }
          frame True {
          }
        }
      }
      frame "Fast Acquire" {
        n129 = local read "Trigger Level (V)"() -> (w360:dbl)
        n130 = local read "Stop Condition"() -> (w363:T2)
        n131 = local read "Range (V)"() -> (w361:dbl)
        n132 = local read "Offset (V)"() -> (w362:dbl)
        n133 = call "InitStopCondition.vi"("Data"=w359, "Stop Condition"=w363, "Offset (V)"=w362, "Range (V)"=w361, "Trigger Level (V)"=w360) -> ("Data Out"=w372:T6)  [unwired: 10 in]
        n134 = case shown="True" "SaveToggle" {
          tunnel: w372 -> [w377 w382]
          tunnel: [w377 w381] -> w355
          tunnel: w354 -> [w376 w380]
          tunnel: [w376 w379] -> w350
          frame False {
          }
          frame True {
            n135 = call "OpenTDMS.vi"("Data In"=w382) -> ("Data Out"=w381:T6)  [unwired: 9 in]
            n136 = Send Notification(notification="Acquisition Start", notifier=w380) -> (notifier out=w379:T4)  [unwired: 1 in, 1 out]
          }
        }
        n137 = flat-sequence {
          tunnel: w355 -> [w383]
          tunnel: [w386] -> w365
          tunnel: [w383] -> w347
          tunnel: w365 -> [w391]
          tunnel: [w391] -> w364
          tunnel: [w388] -> w353
          tunnel: w347 -> [w389]
          frame #0 {
            n138 = local read "Stop Condition"() -> (w385:T2)
            n139 = Unbundle By Name(w383) -> ("DAQ Config Data"=w387:T7)
            n140 = Unbundle By Name(w385) -> ("Duration (S)"=w384:u16)
            n141 = call "AcquisitionFastMode.vi"("Acquisition Time"=w384, "DAQ Config Data"=w387) -> ("Waveforms"=w386:waveform(dbl)[])  [unwired: 9 in]
          }
          frame #1 {
            n142 = Bundle By Name(cluster=w389, "Acquisition.Current.Acquiring Now?"=FALSE) -> (w388:T6)
            n143 = property on="Stop" class="Bool"("DisabledEnum"=T15."Enabled" ("Disabled")) -> ()  [unwired: 2 in, 2 out]
            n144 = call "UpdateUIControls.vi"("Data"=w388) -> ()  [unwired: 11 in]
          }
        }
        n145 = Unbundle By Name(w355) -> ("Acquisition.Current.Acquiring Now?"=w358:bool)
        n146 = control-ref of="Signal"() -> (w367:refnum<vi>)
        n147 = control-ref of="Preliminary Histogram"() -> (w366:refnum<vi>)
        n148 = call "RescaleGraphs.vi"("WaveformGraph in"=w367, "Offset (V) 3"=w362, "Range (V) 3"=w361, "Preliminary Histogram"=w366) -> ()  [unwired: 6 in]
        n149 = local write "Acquiring Now?"(w358) -> ()
        n150 = call "GetandWriteSlowControlData_TDMS.vi"("notifier in"=w350, "queue in"=w352, "Data In"=w353) -> ("notifier out"=w349:T4, "queue out"=w351:T3, "Data Out"=w348:T6)  [unwired: 6 in]
        n151 = Unbundle By Name(w348) -> ("Acquisition.Current.Acquiring Now?"=w357:bool)
        n152 = case shown="True" "SaveToggle" {
          tunnel: w364 -> [_ w374]
          tunnel: w348 -> [_ w373]
          frame False {
          }
          frame True {
            n153 = call "StoreWaveformFastTDMS.vi"("Waveforms"=w374, "Data In"=w373) -> ("tdms file out"=w375:refnum<k34>)  [unwired: 9 in]
            n154 = TDMS Close(11:w375) -> ()  [unwired: 1 in, 2 out]
          }
        }
        n155 = local write "Acquiring Now?"(w357) -> ()
      }
    }
  }
  n156 = Unbundle By Name(w1) -> ("Measurement.TDMS File Handle"=w2:refnum<k34>)
  n157 = TDMS Close(11:w2) -> ()  [unwired: 1 in, 2 out]
